vi "Save File DOE Clean Comments.vi"(11 "Comments: in":string) -> (3 "Comments: out":string)   [LabVIEW 2020, in "File Setup.lvlib"]
uses:
  File Setup.lvlib
  <vilib>/Utility/error.llb/whitespace.ctl
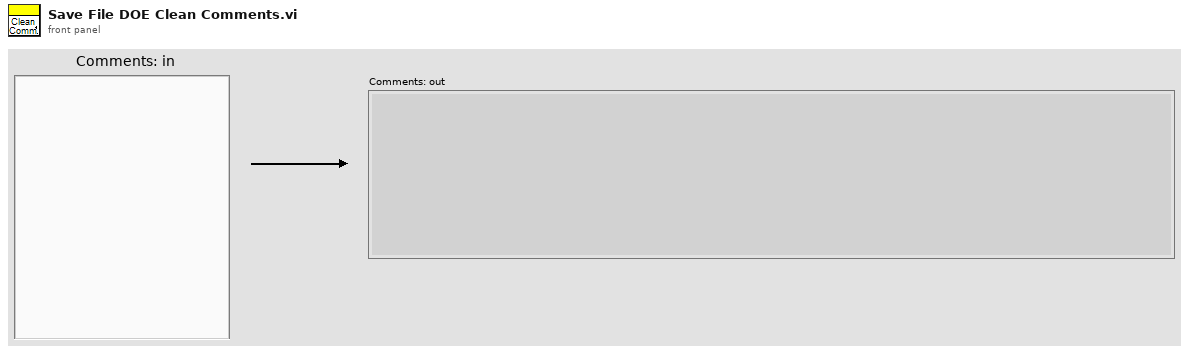
[diagram p1: front panel]
types:
  T1 = typedef "whitespace.ctl" = u16
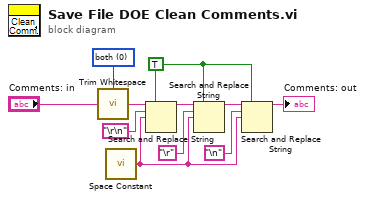
[diagram p0: block diagram]
diagram:
  w4 = TRUE ("replace all? (F)")
  w11 = T1 0 items=["both", "start of string", "end of string"] ("location (both)")
  n1 = call <vilib>:"Trim Whitespace.vi"("string"="Comments: in", "location (both)"=w11) -> ("trimmed string"=w7:string)
  n2 = call <vilib>:"Space Constant.vi"() -> ("String"=w5:string)
  n3 = Search and Replace String(replace all?=w4, input string=w7, search string="\r\n", replace string=w5) -> (result string=w9:string)  [unwired: 4 in, 3 out]
  n4 = Search and Replace String(replace all?=w4, input string=w9, search string="\r", replace string=w5) -> (result string=w3:string)  [unwired: 4 in, 3 out]
  n5 = Search and Replace String(replace all?=w4, input string=w3, search string="\n", replace string=w5) -> (result string=→"Comments: out":string)  [unwired: 4 in, 3 out]
